vi "AutoReloadStateMachine.vi"(11 "Current State In":dbl) -> (3 "Current State Out":dbl)   [LabVIEW 2012]
uses:
  <vilib>/Rock Robotics/WPI/Solenoid/WPI_SolenoidValue.ctl
  Autonomous_Routine_Global.vi
  <vilib>/Rock Robotics/WPI/Joystick/WPI_JoystickGetSetRefNum.vi
  <vilib>/Rock Robotics/WPI/Solenoid/WPI_SolenoidSetEnum.vi
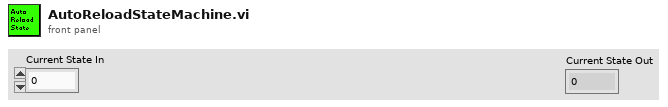
[diagram p1: front panel]
types:
  T1 = typedef "WPI_SolenoidValue.ctl" = enum16{"Off", "On", "Forward", "Reverse"}
  T2 = typedef "WPI_JoystickDevRef.ctl" = cluster{"Device":T3}
  T3 = typedef "WPI_JoystickDeviceEnum.ctl" = enum16{"USB 1", "USB 2", "USB 3", "USB 4", "Kinect 1", "Kinect 2"}
  T4 = typedef "WPI_JoystickButtonState.ctl" = cluster{"Button 1":bool, "Button 2":bool, "Button 3":bool, "Button 4":bool, "Button 5":bool, "Button 6":bool, "Button 7":bool, "Button 8":bool, "Button 9":bool, "Button 10":bool, "Button 11":bool, "Button 12":bool}
  T5 = cluster{"axis 1 (x)":dbl, "axis 2 (y)":dbl, "axis 3 (throttle)":dbl, "axis 4":dbl, "axis 5":dbl, "axis 6":dbl}
  T6 = typedef "WPI_SolenoidDevRef.ctl" = cluster{"DevStatus":errorcluster, "Solenoid Module":T7, "Forward Solenoid Channel":T8, "Reverse Solenoid Channel":T8}
  T7 = typedef "FPGA_TypedefSolenoidModule.ctl" = enum16{"Solenoid Module 1", "Solenoid Module 2"}
  T8 = typedef "WPI_SolenoidChannel.ctl" = enum8{"Solenoid 1", "Solenoid 2", "Solenoid 3", "Solenoid 4", "Solenoid 5", "Solenoid 6", "Solenoid 7", "Solenoid 8", "Invalid"}
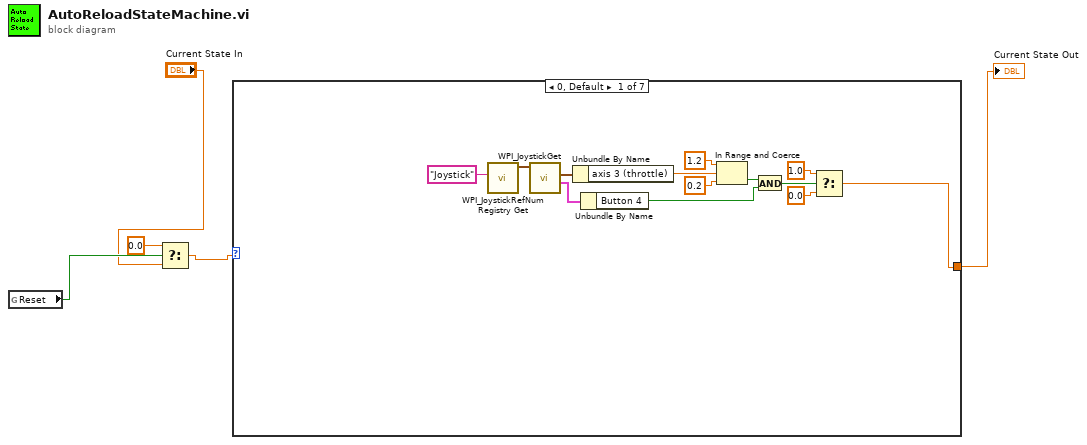
[diagram p0: block diagram]
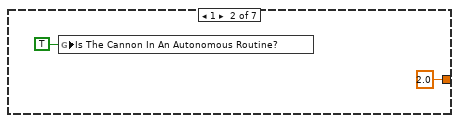
[diagram p2: hidden frame]
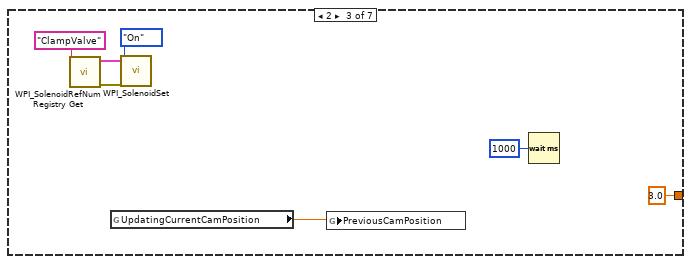
[diagram p3: hidden frame]
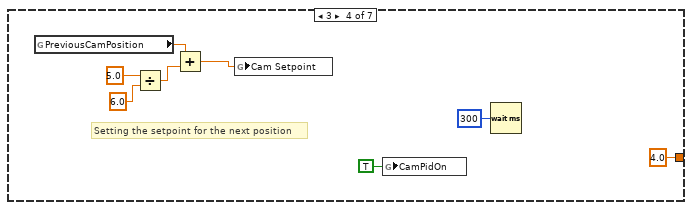
[diagram p4: hidden frame]
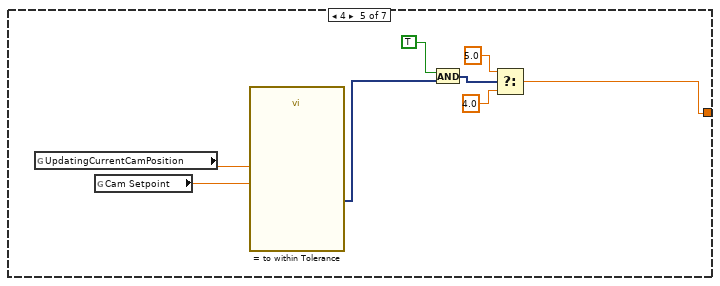
[diagram p5: hidden frame]
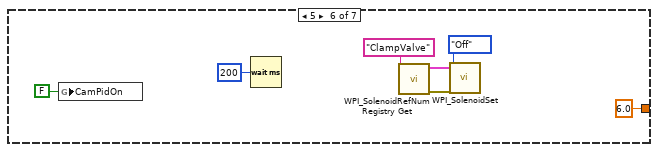
[diagram p6: hidden frame]
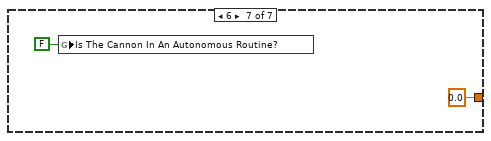
[diagram p7: hidden frame]
diagram:
  n1 = global read "Autonomous_Routine_Global.vi" "Reset"() -> (w4:bool)
  n2 = Select(t=0.0, s=w4, f="Current State In") -> (s? t:f=w2:dbl)
  n3 = case shown="0, Default" w2 {
    tunnel: [w6 2.0 ("t") 3.0 ("t") 4.0 ("t") w41 6.0 ("f") 0.0 ("f")] -> w5
    frame 0, Default {
      n4 = call <vilib>:"WPI_JoystickRefNum Registry Get.vi"("refnum name"="Joystick") -> ("JoystickDevRef"=w18:T2)  [unwired: 9 in, 1 out]
      n5 = call <vilib>:"WPI_JoystickGet.vi"("JoystickDevRef"=w18) -> ("Buttons"=w11:T4, "Axes"=w16:T5)  [unwired: 4 in, 1 out]
      n6 = Unbundle By Name(w16) -> ("axis 3 (throttle)"=w15:dbl)
      n7 = Unbundle By Name(w11) -> ("Button 4"=w10:bool)
      n8 = In Range and Coerce(upper limit=1.2, x=w15, lower limit=0.2 ("upper limit")) -> (In Range?=w12:bool)  [unwired: 1 out]
      n9 = And(x=w12, y=w10) -> (x .and. y?=w9:bool)
      n10 = Select(t=1.0, s=w9, f=0.0 ("t")) -> (s? t:f=w6:dbl)
    }
    frame 1 {
      n11 = global write "Autonomous_Routine_Global.vi" "Is The Cannon In An Autonomous Routine?"(TRUE ("Is The Cannon In An Autonomous Routine?")) -> ()
    }
    frame 2 {
      n12 = call <vilib>:"WPI_SolenoidRefNum Registry Get.vi"("refnum name"="ClampValve") -> ("error out"=w27:errorcluster, "SolenoidDevRef"=w26:T6)  [unwired: 9 in]
      n13 = global read "Autonomous_Routine_Global.vi" "UpdatingCurrentCamPosition"() -> (w21:dbl)
      n14 = call-poly <vilib>:"WPI_SolenoidSet.vi"("error in (no error)"=w27, "Value"=WPI_SolenoidValue."On", "SolenoidDevRef"=w26) -> ()  [unwired: 7 in, 2 out]
      n15 = global write "Autonomous_Routine_Global.vi" "PreviousCamPosition"(w21) -> ()
      n16 = Wait (ms)(milliseconds to wait=u32 1000) -> ()  [unwired: 1 out]
    }
    frame 3 {
      # "Setting the setpoint for the next position"
      n17 = global read "Autonomous_Routine_Global.vi" "PreviousCamPosition"() -> (w32:dbl)
      n18 = Divide(x=5.0, y=6.0) -> (x/y=w31:dbl)
      n19 = Add(x=w32, y=w31) -> (x+y=w28:dbl)
      n20 = global write "Autonomous_Routine_Global.vi" "Cam Setpoint"(w28) -> ()
      n21 = global write "Autonomous_Routine_Global.vi" "CamPidOn"(TRUE ("CamPidOn")) -> ()
      n22 = Wait (ms)(milliseconds to wait=u32 300) -> ()  [unwired: 1 out]
    }
    frame 4 {
      n23 = global read "Autonomous_Routine_Global.vi" "UpdatingCurrentCamPosition"() -> (w39:dbl)
      n24 = global read "Autonomous_Routine_Global.vi" "Cam Setpoint"() -> (w38:dbl)
      n25 = call "= to within Tolerance"("Operand 2"=w38, "Operand 1"=w39) -> ("Result"=w37:dynamicdata)  [unwired: 8 in, 1 out]
      n26 = And(x=TRUE, y=w37) -> (x .and. y?=w40:dynamicdata)
      n27 = Select(t=5.0, s=w40, f=4.0) -> (s? t:f=w41:dbl)
    }
    frame 5 {
      n28 = global write "Autonomous_Routine_Global.vi" "CamPidOn"(FALSE ("CamPidOn")) -> ()
      n29 = Wait (ms)(milliseconds to wait=u32 200) -> ()  [unwired: 1 out]
      n30 = call <vilib>:"WPI_SolenoidRefNum Registry Get.vi"("refnum name"="ClampValve") -> ("error out"=w49:errorcluster, "SolenoidDevRef"=w48:T6)  [unwired: 9 in]
      n31 = call-poly <vilib>:"WPI_SolenoidSet.vi"("error in (no error)"=w49, "Value"=WPI_SolenoidValue."Off", "SolenoidDevRef"=w48) -> ()  [unwired: 7 in, 2 out]
    }
    frame 6 {
      n32 = global write "Autonomous_Routine_Global.vi" "Is The Cannon In An Autonomous Routine?"(FALSE ("Is The Cannon In An Autonomous Routine?")) -> ()
    }
  }
  "Current State Out" <- w5
